vi "Add to write queue.vi"(8 "error in (no error)":errorcluster, 10 "Write item":T1, 11 "WAMP Client in":refnum<class "WAMP Client.lvclass">) -> (0 "error out":errorcluster)   [LabVIEW 2020, in "wamplv.lvlib" / "WAMP Client.lvclass"]
uses:
  WAMP Client.lvclass
  WAMP Client.lvclass/WAMP Client.ctl
  Private/TypeDefs/Transport type.ctl
  wamplv.lvlib
  TypeDef/Write queue item.ctl
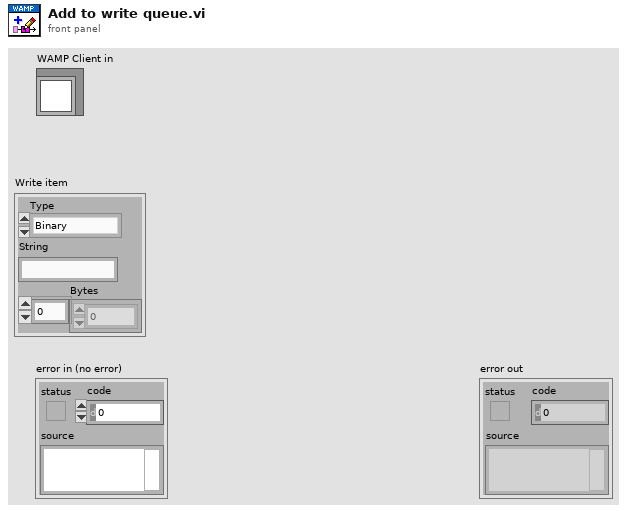
[diagram p1: front panel]
types:
  T1 = typedef "wamplv.lvlib/Write queue item.ctl" = cluster{"Type":T2, "String":string, "Bytes":u8[]}
  T2 = typedef "wamplv.lvlib/Transport type.ctl" = enum16{"Binary", "Text"}
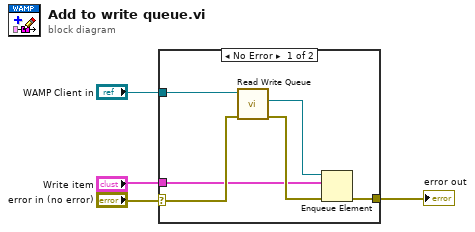
[diagram p0: block diagram]
diagram:
  n1 = case shown="No Error" "error in (no error)" {
    selector: "error in (no error)" -> [w6 w11]
    tunnel: [w10 w11] -> w3
    tunnel: "WAMP Client in" -> [w9 _]
    tunnel: "Write item" -> [w5 _]
    frame No Error {
      n2 = call "Read Write Queue.vi"("error in (no error)"=w6, "WAMP Client in"=w9) -> ("error out"=w7:errorcluster, "Write Queue"=w8:refnum<queue>)  [unwired: 7 in, 1 out]
      n3 = Enqueue Element(queue=w8, element=w5, error in (no error)=w7) -> (error out=w10:errorcluster)  [unwired: 1 in, 2 out]
    }
    frame Error {
    }
  }
  "error out" <- w3
